vi "Weather Station UI.vi"(7 "정지":bool, 9 "하위 리미트":dbl=10.0 min=0.0 max=50.0, 10 "상위 리미트":dbl=30.0 min=0.0 max=50.0) -> (1 "경고":string, 2 "온도 히스토리":dbl(graph))   [LabVIEW 2010]
doc: "이 VI는 기상 관측기 프로젝트의 주요 VI입니다. 온도 경고 시스템을 위한 사용자 인터페이스를 포함합니다. 매 0.5초마다 온도를 측정하고, 경고가 발생할 때 데이터를 로그합니다.\n\n사용자 입력: 온도 상위 리미트, 온도 하위 리미트, 온도 단위."
uses:
  Supporting Files/Weather Station States.ctl
panel:
  in  "풍속 상위 리미트":dbl(slide)=50.0 scale=0.0..100.0
  out "풍속 히스토리":dbl(graph)
  in  "날씨 데이터":dynamicdata(graph)
  # "섭씨"
  # "온도 범위 (C)"
  # "열사병"
  # "동상"
  # "kph"
  # "최대 안전 풍속 (kph)"
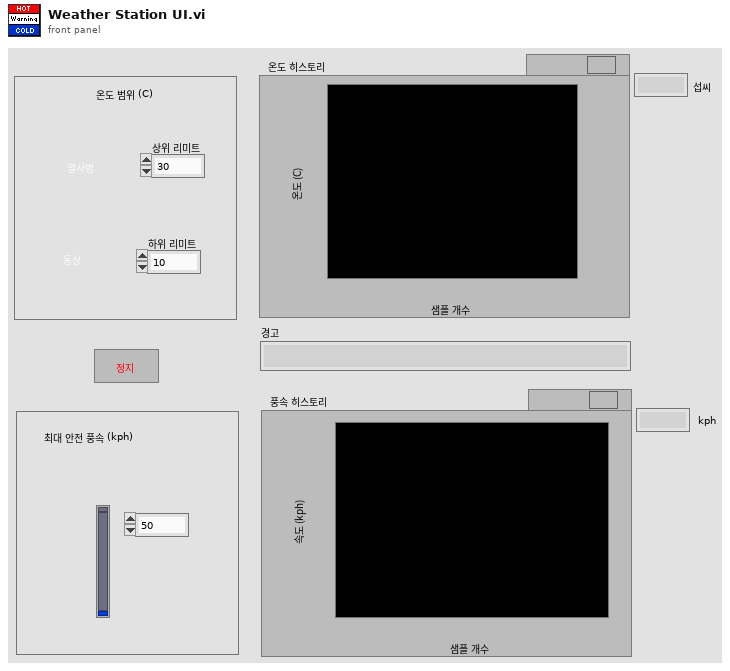
[diagram p1: front panel]
types:
  T1 = cluster{"온도":dbl, "온도 상위 리미트":dbl, "온도 하위 리미트":dbl, "풍속":dbl, "풍속 상위 리미트":dbl, "경고":string, "시간":dbl}
  T2 = typedef "Weather Station States.ctl" = enum16{"분석", "UI 처리", "경고 설정", "데이터 로그", "정지"}
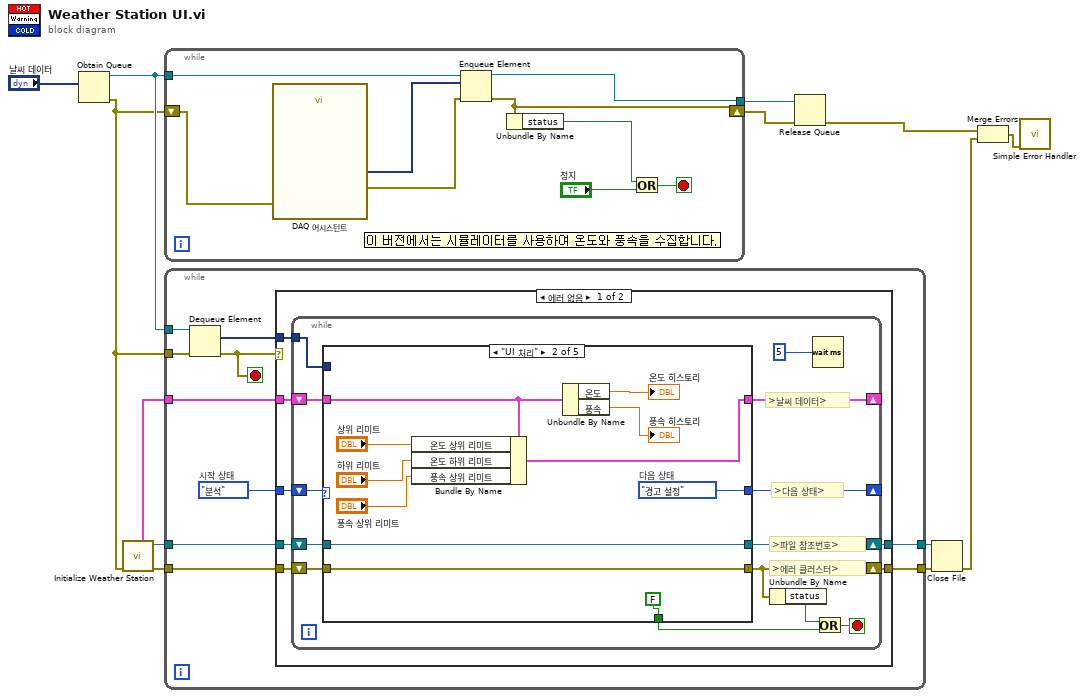
[diagram p0: block diagram]
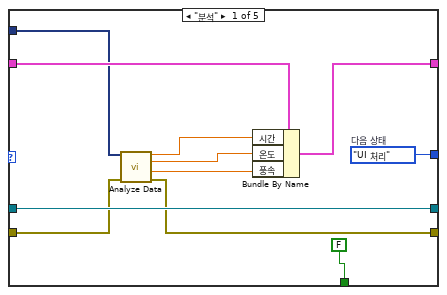
[diagram p2: hidden frame]
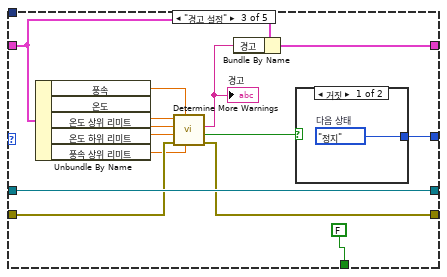
[diagram p3: hidden frame]
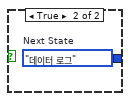
[diagram p4: hidden frame]
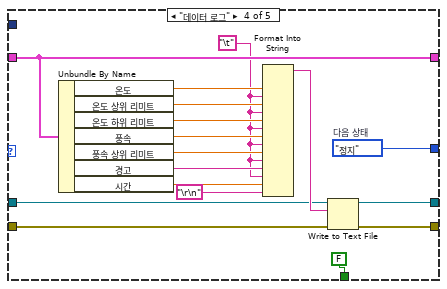
[diagram p5: hidden frame]
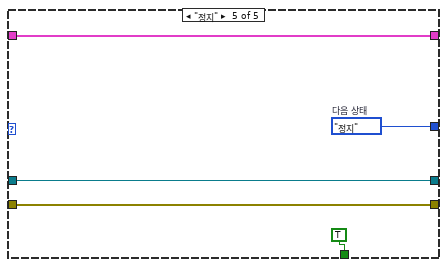
[diagram p6: hidden frame]
diagram:
  n1 = Obtain Queue(element data type="날씨 데이터") -> (queue out=w5:refnum<queue>, error out=w1:errorcluster)  [unwired: 3 in, 2 out]
  n2 = call "Initialize Weather Station.vi"("에러 입력(에러 없음)"=w1) -> ("에러 출력"=w10:errorcluster, "파일 참조 번호"=w11:refnum<file>, "날씨 데이터"=w9:T1)  [unwired: 8 out]
  n3 = while {
    tunnel: w5 -> [w22]
    tunnel: [w21] -> w7
    shift-right: [w18] -> w6
    shift-left: w1 -> [w16]
    stop <- w20 stop-if-true
    n4 = call "DAQ 어시스턴트"("error in"=w16) -> ("data"=w14:dynamicdata, "error out"=w15:errorcluster)  [unwired: 16 in, 1 out]
    n5 = Enqueue Element(queue=w22, element=w14, error in (no error)=w15) -> (queue out=w21:refnum<queue>, error out=w18:errorcluster)  [unwired: 2 out]
    n6 = Unbundle By Name(w18) -> ("status"=w17:bool)
    n7 = Or(x=w17, y="정지") -> (x .or. y?=w20:bool)
  }
  n8 = while {
    tunnel: [w31] -> w13
    tunnel: [w30] -> w12
    tunnel: w11 -> [w29]
    tunnel: w10 -> [w28]
    tunnel: w9 -> [w27]
    tunnel: w5 -> [w26]
    tunnel: w1 -> [w25]
    stop <- w24 stop-if-true
    w32 = Weather_Station_States."분석"  # 시작 상태
    n9 = Dequeue Element(queue=w26, error in (no error)=w25) -> (element=w23:dynamicdata, error out=w24:errorcluster)  [unwired: 3 out]
    n10 = case shown="에러 없음" w24 {
      tunnel: w32 -> [w39 _]
      tunnel: [w38 w113] -> w31
      tunnel: [w37 w114] -> w30
      tunnel: w29 -> [w36 w114]
      tunnel: w28 -> [w35 w113]
      tunnel: w27 -> [w34 _]
      tunnel: w23 -> [w33 _]
      frame No Error {
        n11 = while {
          shift-right: [w51] -> _
          shift-left: w39 -> [w52]
          shift-right: [w48] -> w38
          shift-left: w35 -> [w50]
          shift-right: [w41] -> _
          shift-left: w34 -> [w45]
          shift-right: [w46] -> w37
          shift-left: w36 -> [w44]
          tunnel: w33 -> [w40]
          stop <- w49 stop-if-true
          # ">에러 클러스터>"
          # ">날씨 데이터>"
          # ">파일 참조번호>"
          # ">다음 상태>"
          n12 = case shown="\"UI 처리\"" w52 {
            tunnel: [w63 w65 w86 w107 w108] -> w51
            tunnel: [w56 w66 w79 w105 w110] -> w48
            tunnel: w50 -> [w58 w66 w80 w106 w110]
            tunnel: [w62 w67 w88 w104 w111] -> w46
            tunnel: [w59 w71 w81 w96 w112] -> w41
            tunnel: w45 -> [w60 w72 w82 w96 w112]
            tunnel: w44 -> [w62 w67 w88 w102 w111]
            tunnel: [FALSE ("stop") FALSE ("stop") FALSE ("stop") FALSE ("stop") TRUE ("stop")] -> w43
            tunnel: w40 -> [w57 _ _ _ _]
            frame "분석" {
              w63 = Weather_Station_States."UI 처리"  # 다음 상태
              n13 = call "Analyze Data.vi"("날씨 데이터"=w57, "에러 입력"=w58) -> ("시간"=w55:dbl, "온도"=w54:dbl, "풍속"=w53:dbl, "에러 출력"=w56:errorcluster)  [unwired: 10 out]
              n14 = Bundle By Name(cluster=w60, "시간"=w55, "온도"=w54, "풍속"=w53) -> (w59:T1)
            }
            frame "UI 처리" {
              w65 = Weather_Station_States."경고 설정"  # 다음 상태
              n15 = Bundle By Name(cluster=w72, "온도 상위 리미트"="상위 리미트", "온도 하위 리미트"="하위 리미트", "풍속 상위 리미트"="풍속 상위 리미트") -> (w71:T1)
              n16 = Unbundle By Name(w72) -> ("온도"=→"온도 히스토리":dbl, "풍속"=→"풍속 히스토리":dbl)
            }
            frame "경고 설정" {
              n17 = Unbundle By Name(w82) -> ("풍속"=w76:dbl, "온도"=w85:dbl, "온도 상위 리미트"=w84:dbl, "온도 하위 리미트"=w83:dbl, "풍속 상위 리미트"=w75:dbl)
              n18 = call "Determine More Warnings.vi"("최대 풍속"=w75, "현재 풍속"=w76, "에러 입력(에러 없음)"=w80, "최저 온도"=w83, "최고 온도"=w84, "현재 온도"=w85) -> ("에러 출력"=w79:errorcluster, "경고?"=w77:bool, "경고 텍스트"=w78:string)  [unwired: 3 out]
              "경고" <- w78
              n19 = Bundle By Name(cluster=w82, "경고"=w78) -> (w81:T1)
              n20 = case shown="거짓" w77 {
                tunnel: [w89 w90] -> w86
                frame False {
                  w89 = Weather_Station_States."정지"  # 다음 상태
                }
                frame True {
                  w90 = Weather_Station_States."데이터 로그"  # Next State
                }
              }
            }
            frame "데이터 로그" {
              w107 = Weather_Station_States."정지"  # 다음 상태
              w93 = "\t" ("Tab Constant")
              n21 = Unbundle By Name(w96) -> ("온도"=w100:dbl, "온도 상위 리미트"=w99:dbl, "온도 하위 리미트"=w98:dbl, "풍속"=w97:dbl, "풍속 상위 리미트"=w95:dbl, "경고"=w94:string, "시간"=w92:dbl)
              n22 = Format Into String(w100, w93, w99, w93, w98, w93, w97, w93, w95, w93, w94, w93, w92, "\r\n" ("End of Line Constant")) -> (resulting string=w103:string)  [unwired: 3 in, 1 out]
              n23 = Write to Text File(file (use dialog)=w102, text=w103, error in=w106) -> (refnum out=w104:refnum<file>, error out=w105:errorcluster)  [unwired: 2 out]
            }
            frame "정지" {
              w108 = Weather_Station_States."정지"  # 다음 상태
            }
          }
          n24 = Unbundle By Name(w48) -> ("status"=w47:bool)
          n25 = Wait (ms)(milliseconds to wait=u32 5 ("y")) -> ()  [unwired: 1 out]
          n26 = Or(x=w47, y=w43) -> (x .or. y?=w49:bool)
        }
      }
      frame Error {
      }
    }
  }
  n27 = Release Queue(queue=w7, error in (no error)=w6) -> (error out=w4:errorcluster)  [unwired: 3 out]
  n28 = Close File(refnum=w12, error in=w13) -> (error out=w3:errorcluster)  [unwired: 1 out]
  n29 = Merge Errors(w4, w3) -> (w2:errorcluster)
  n30 = call <vilib>:"Simple Error Handler.vi"("error in (no error)"=w2) -> ()  [unwired: 1 in, 8 out]
